vi "Initialize-message-queues.vi"(8 "error in (no error)":errorcluster, 11 "Object ref in":T1) -> (0 "error out":errorcluster, 3 "Object ref out":T1)   [LabVIEW 2013, in "SLMControl.lvlib" / "SC-Main.lvclass"]
uses:
  SC-Main.lvclass
  Object-reference.ctl
  Deposition-actions.ctl
  Main-actions.ctl
  Lasing-actions.ctl
  SC-Main.lvclass/SC-Main.ctl
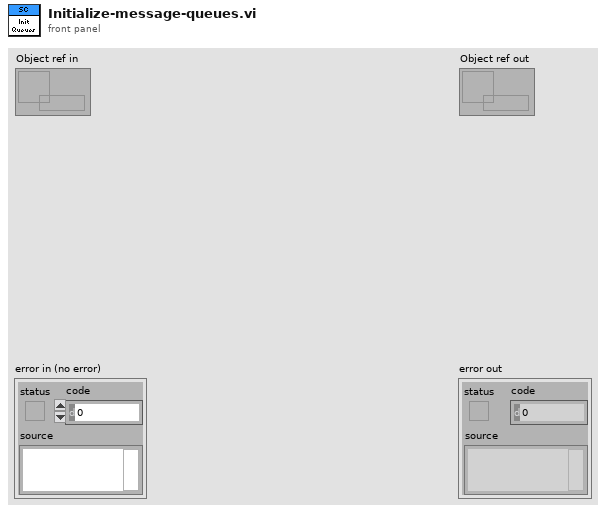
[diagram p1: front panel]
types:
  T1 = typedef "SLMControl.lvlib/SC-Main.lvclass/Object-reference.ctl" = refnum<data-value>
  T2 = typedef "SLMControl.lvlib/SC-Main.lvclass/Lasing-actions.ctl" = enum16{"Idle", "Activate", "Load lasing file", "Launch lasing", "Wait for lasing end", "Signal iterate", "Signal abort", "Abort", "Reset", "Exit"}
  T3 = typedef "SLMControl.lvlib/SC-Main.lvclass/Main-actions.ctl" = enum16{"Idle", "Initialize", "Load configuration", "Save configuration", "Load lasing files", "Load deposition files", "Refresh files", "Clear files", "Open lasing file", "Activate", "Start", "Start deposition cycle", "Start lasing cycle", "Iterate", "Abort", "Stop", "Exit"}
  T4 = typedef "SLMControl.lvlib/SC-Main.lvclass/Deposition-actions.ctl" = enum16{"Idle", "Activate", "Load deposition", "Launch deposition", "Wait for deposition end", "Signal lasing", "Abort", "Reset", "Exit"}
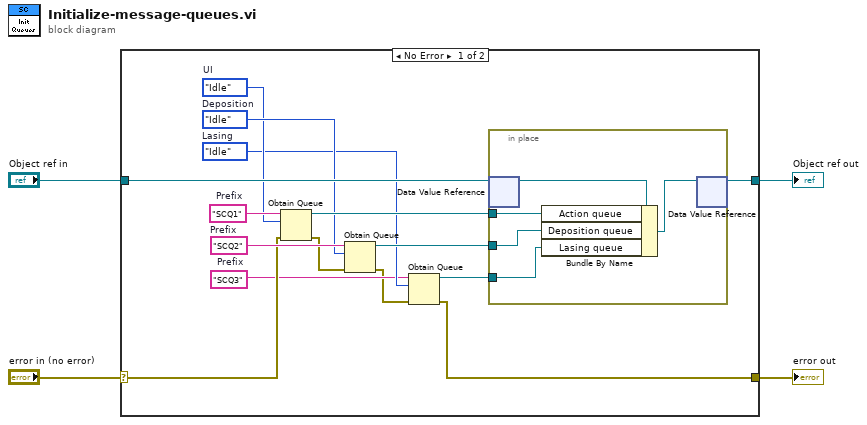
[diagram p0: block diagram]
diagram:
  n1 = case shown="No Error" "error in (no error)" {
    selector: "error in (no error)" -> [w14 w26]
    tunnel: [w6 w26] -> w3
    tunnel: [w18 w25] -> w1
    tunnel: "Object ref in" -> [w19 w25]
    frame No Error {
      w9 = Lasing-actions."Idle"  # Lasing
      w8 = "SCQ3"  # Prefix
      w10 = Main-actions."Idle"  # UI
      w11 = Deposition-actions."Idle"  # Deposition
      w16 = "SCQ2"  # Prefix
      w15 = "SCQ1"  # Prefix
      n2 = Obtain Queue(name (unnamed)=w15, element data type=w10, error in (no error)=w14) -> (queue out=w12:refnum<queue>, error out=w13:errorcluster)  [unwired: 2 in, 1 out]
      n3 = Obtain Queue(name (unnamed)=w16, element data type=w11, error in (no error)=w13) -> (queue out=w17:refnum<queue>, error out=w7:errorcluster)  [unwired: 2 in, 1 out]
      n4 = Obtain Queue(name (unnamed)=w8, element data type=w9, error in (no error)=w7) -> (queue out=w5:refnum<queue>, error out=w6:errorcluster)  [unwired: 2 in, 1 out]
      n5 = in-place {
        in-place-border: w12 -> [w22]
        in-place-border: w17 -> [w21]
        in-place-border: w5 -> [w20]
        n6 = in-place-dvr #1(w19) -> (w24:refnum<class "SC-Main.lvclass">)  [unwired: 1 out]
        n7 = Bundle By Name(cluster=w24, "Action queue"=w22, "Deposition queue"=w21, "Lasing queue"=w20) -> (w23:refnum<class "SC-Main.lvclass">)
        n8 = in-place-dvr #1(w23) -> (w18:T1)  [unwired: 1 out]
      }
    }
    frame Error {
    }
  }
  "error out" <- w3
  "Object ref out" <- w1
